vi "AbortSub.vi"(9 "aborted":bool, 11 "SubChannel in":refnum<class "SubChannelCPU.lvclass">) -> (3 "SubChannel out":refnum<class "SubChannelCPU.lvclass">)   [LabVIEW 2019, in "MessengerM.lvlib" / "SubChannelCPU.lvclass"]
uses:
  SubChannelCPU.lvclass
  <resource>/ChannelSupport/_ChannelSupport/PipeLogic2/PipeLogic2.lvclass
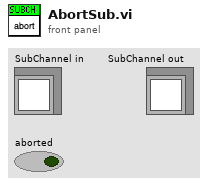
[diagram p1: front panel]
types:
  T1 = typedef "MessengerM.lvlib/Element.ctl" = string
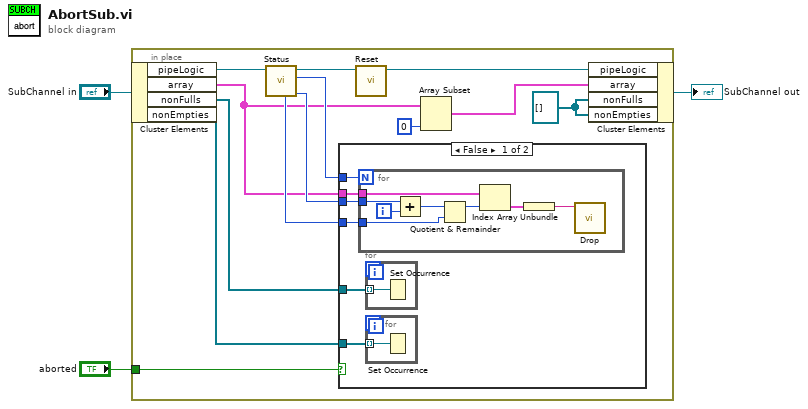
[diagram p0: block diagram]
diagram:
  n1 = in-place {
    in-place-border: "aborted" -> [w10]
    w7 = refnum<k4>[] [] ("nonFulls")
    n2 = in-place-cluster #1("SubChannel in") -> ("pipeLogic"=w12:refnum<class "PipeLogic2.lvclass">, "array"=w5:cluster{"elt":T1}[], "nonFulls"=w9:refnum<k4>[], "nonEmpties"=w8:refnum<k4>[])
    n3 = call <resource>:"Status.vi"("pipeLogic in"=w12) -> ("index out"=w15:i32, "count"=w16:i32, "pipeLogic out"=w13:refnum<class "PipeLogic2.lvclass">, "size"=w14:i32)  [unwired: 4 in, 3 out]
    n4 = case shown="False" w10 {
      tunnel: w16 -> [w22 _]
      tunnel: w15 -> [w20 _]
      tunnel: w14 -> [w19 _]
      tunnel: w5 -> [w21 _]
      tunnel: w9 -> [w18 _]
      tunnel: w8 -> [w17 _]
      frame False {
        n5 = for {
          N: w22 -> [_]
          tunnel: w21 -> [w32]
          tunnel: w20 -> [w31]
          tunnel: w19 -> [w27]
          i -> [w30]
          n6 = Add(x=w31, y=w30) -> (x+y=w29:i32)
          n7 = Quotient & Remainder(x=w29, y=w27) -> (x-y*floor(x/y)=w28:i32)  [unwired: 1 out]
          n8 = Index Array(array=w32, index=w28) -> (element=w26:cluster{"elt":T1})
          n9 = Unbundle(w26) -> ("elt"=w25:T1)
          n10 = call "Drop.vi"("element in"=w25) -> ()  [unwired: 11 in]
        }
        n11 = for {
          tunnel: w18 -> [w24] mode=indexing
          n12 = Set Occurrence(w24) -> ()
        }
        n13 = for {
          tunnel: w17 -> [w23] mode=indexing
          n14 = Set Occurrence(w23) -> ()
        }
      }
      frame True {
      }
    }
    n15 = call <resource>:"Reset.vi"("pipeLogic in"=w13) -> ("pipeLogic out"=w11:refnum<class "PipeLogic2.lvclass">)  [unwired: 10 in]
    n16 = Array Subset(array=w5, length=0) -> (w6:cluster{"elt":T1}[])  [unwired: 1 in]
    n17 = in-place-cluster #1("pipeLogic"=w11, "array"=w6, "nonFulls"=w7, "nonEmpties"=w7) -> (→"SubChannel out":refnum<class "SubChannelCPU.lvclass">)
  }
